vi "Button State Get.vi"(8 "error in (no error)":errorcluster) -> (0 "error out":errorcluster, 2 "Button State":bool)   [LabVIEW 2019, in "Haptic Prog Interface.lvlib"]
doc: "Returns the button state of the haptic pen.\n\n<b>Button State:</b> Returns the boolean state of the pen button."
uses:
  Haptic Prog Interface.lvlib
  dll_path.vi
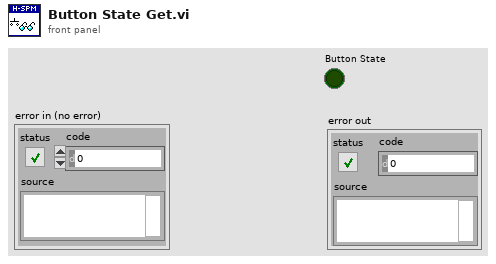
[diagram p1: front panel]
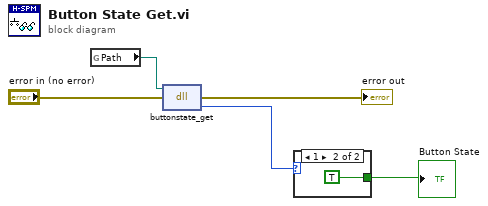
[diagram p0: block diagram]
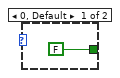
[diagram p2: hidden frame]
diagram:
  n1 = global read "dll_path.vi" "Path"() -> (w5:path)
  n2 = dll-call lib="C:/Users/freem/Documents/GitHub/HapticSPM/Haptic-Programming-Interface/x64/Debug/Haptic Programming Interface.dll" fn="buttonstate_get"(path in=w5, error in="error in (no error)") -> (error out=→"error out":errorcluster, "return type"=w2:i8)  [unwired: 1 in, 1 out]
  n3 = case shown="1" w2 {
    tunnel: [FALSE TRUE] -> w1
    frame 0, Default {
    }
    frame 1 {
    }
  }
  "Button State" <- w1
